vi "HEWH Draw Logic.vi"(6 "PRAT?":bool, 8 "Error In":errorcluster, 9 "Skip Purge in":bool, 10 "Skip Draw in":bool, 11 "Skip Draw And Purge":bool) -> (0 "Error Out":errorcluster, 1 "Skip Purge out":bool, 2 "Skip Valve Setup":bool, 3 "Skip Draw out":bool)   [LabVIEW 2016]
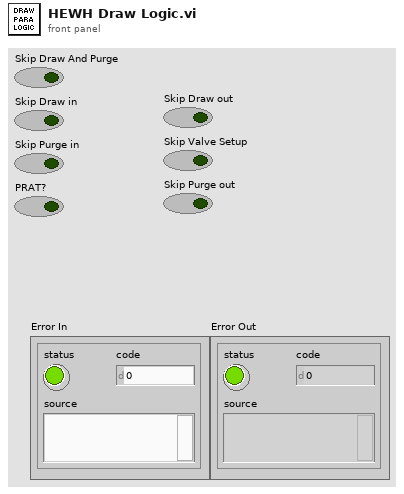
[diagram p1: front panel]
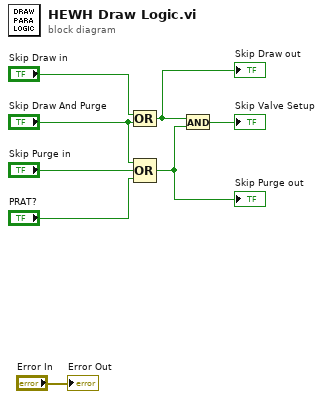
[diagram p0: block diagram]
diagram:
  n1 = Compound Arithmetic op=OR("Skip Draw in", "Skip Draw And Purge") -> (w4:bool)
  "Skip Draw out" <- w4
  n2 = Compound Arithmetic op=OR("Skip Draw And Purge", "Skip Purge in", "PRAT?") -> (w3:bool)
  "Skip Purge out" <- w3
  n3 = And(x=w4, y=w3) -> (x .and. y?=→"Skip Valve Setup":bool)
  "Error Out" <- "Error In"
